vi "(25) part 2 que.vi"() -> ()   [LabVIEW 2025]
panel:
  out "x*y":i32
  out "x+y":i32
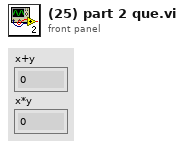
[diagram p1: front panel]
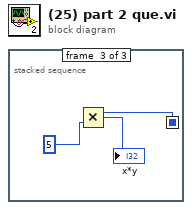
[diagram p0: block diagram]
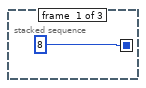
[diagram p2: hidden frame]
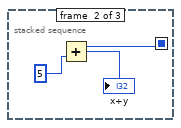
[diagram p3: hidden frame]
diagram:
  n1 = stacked-sequence {
    seq-local: [8 _ _] -> [_ w3 w6]
    frame #0 {
    }
    frame #1 {
      n2 = Add(x=w3, y=5) -> (x+y=→"x+y":i32)
    }
    frame #2 {
      n3 = Multiply(x=w6, y=5) -> (x*y=→"x*y":i32)
    }
  }
